vi "nonlinear spring rhs.vi"(2 "data":variant, 3 "t":dbl, 4 "x":dbl[](array[numeric])) -> (0 "error out":errorcluster, 1 "f(x,t)":dbl[](array[numeric]))   [LabVIEW 2023]
doc: "Create the nonlinear spring function that is the right-hand-side of an ordinary differential equation to be passed to the ODE Solver.vi."
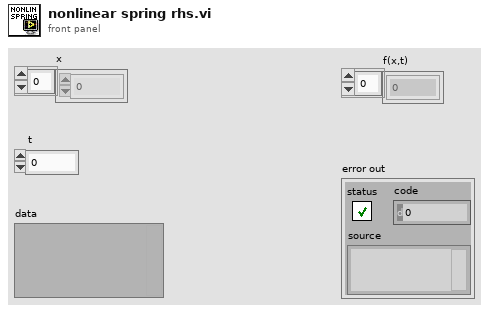
[diagram p1: front panel]
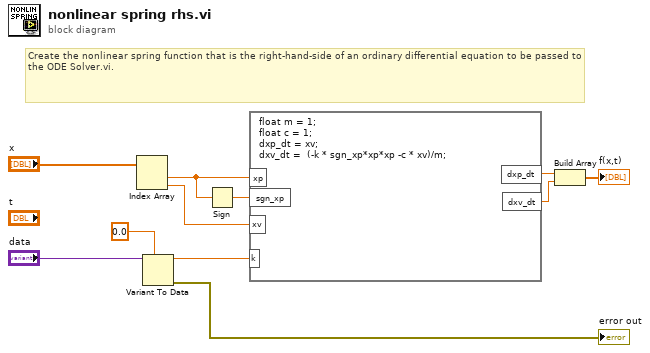
[diagram p0: block diagram]
diagram:
  # "Create the nonlinear spring function that is the right-hand-side of an ordinary differential equation to be passed to the ODE Solver.vi."
  n1 = Index Array(array="x") -> (element #1=w4:dbl, element #2=w10:dbl)  [unwired: 2 in]
  n2 = Variant To Data(type=0.0 ("element"), Variant="data") -> (data=w5:dbl, error out=→"error out":errorcluster)  [unwired: 1 in]
  n3 = Sign(1:w4) -> (0:w3:dbl)
  n4 = formula code="float m = 1;\nfloat c = 1;\ndxp_dt = xv;\ndxv_dt =  (-k * sgn_xp*xp*xp -c * xv)/m;"("xp"=w4, "xv"=w10, "k"=w5, "sgn_xp"=w3) -> ("dxp_dt"=w9:dbl, "dxv_dt"=w1:dbl)
  n5 = Build Array(w9, w1) -> (→"f(x,t)":dbl[])
